vi "Read Data.vi"(8 "error in (no error)":errorcluster, 11 "Single in":refnum<class "Single.lvclass">) -> (0 "error out":errorcluster, 2 "Data":sgl, 3 "Single out":refnum<class "Single.lvclass">)   [LabVIEW 2018, in "Base Data Class.lvlib" / "Single.lvclass"]
uses:
  Single.lvclass
  Single.lvclass/Single.ctl
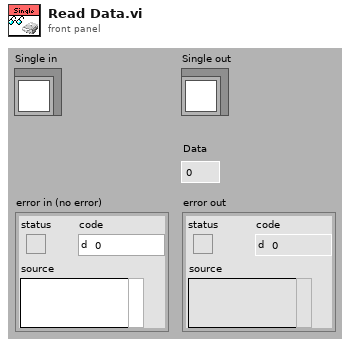
[diagram p1: front panel]
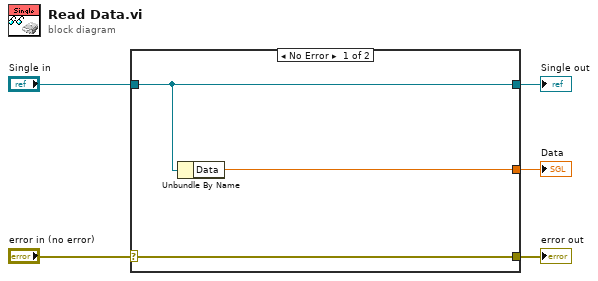
[diagram p0: block diagram]
diagram:
  n1 = case shown="No Error" "error in (no error)" {
    selector: "error in (no error)" -> [w8 w9]
    tunnel: [w8 w9] -> w4
    tunnel: [w7 w10] -> w2
    tunnel: "Single in" -> [w7 w10]
    tunnel: [w6 _] -> w1
    frame No Error {
      n2 = Unbundle By Name(w7) -> ("Data"=w6:sgl)
    }
    frame Error {
    }
  }
  "error out" <- w4
  "Single out" <- w2
  "Data" <- w1
